vi "ZC_biaoqian.vi"(7 "LabVIEW Web Service Request":refnum<class "Web Request.lvclass"> caption="LabVIEW Web服务请求", 8 "key":string, 9 "number":string, 10 "action":string, 11 "id":string) -> (6 "error":errorcluster)   [LabVIEW 2017]
uses:
  <vilib>/wsapi/Web Request.lvclass
panel:
  out "postdata":string caption="post数据"
  out "error out":errorcluster caption="错误输出"
  # "Web服务请求输入接线端用于调用“Web服务”选板的VI。除非不需要访问该选板，否则不要在连线板上删除这个输入接线端。"
  # "添加至连线板的每一个其他输入控件，在URL中对应于一个输入。如需在接线端模式输出（默认设置）下包含显示控件，则该显示控件必须与连线板相连。"
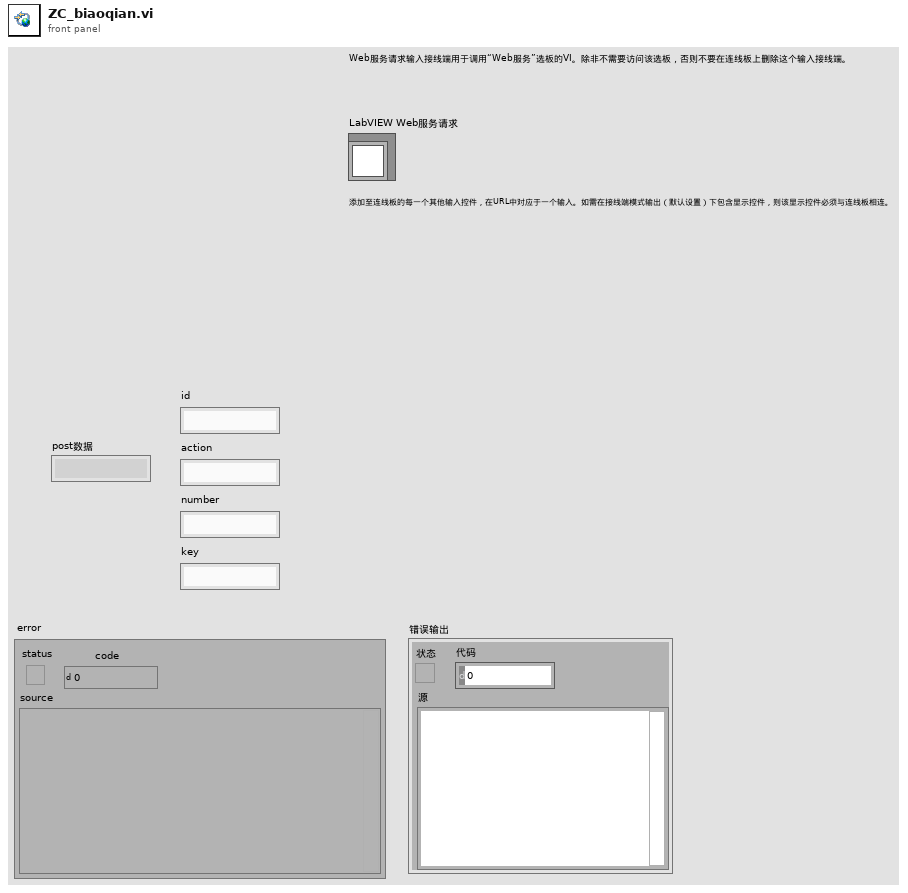
[diagram p1: front panel]
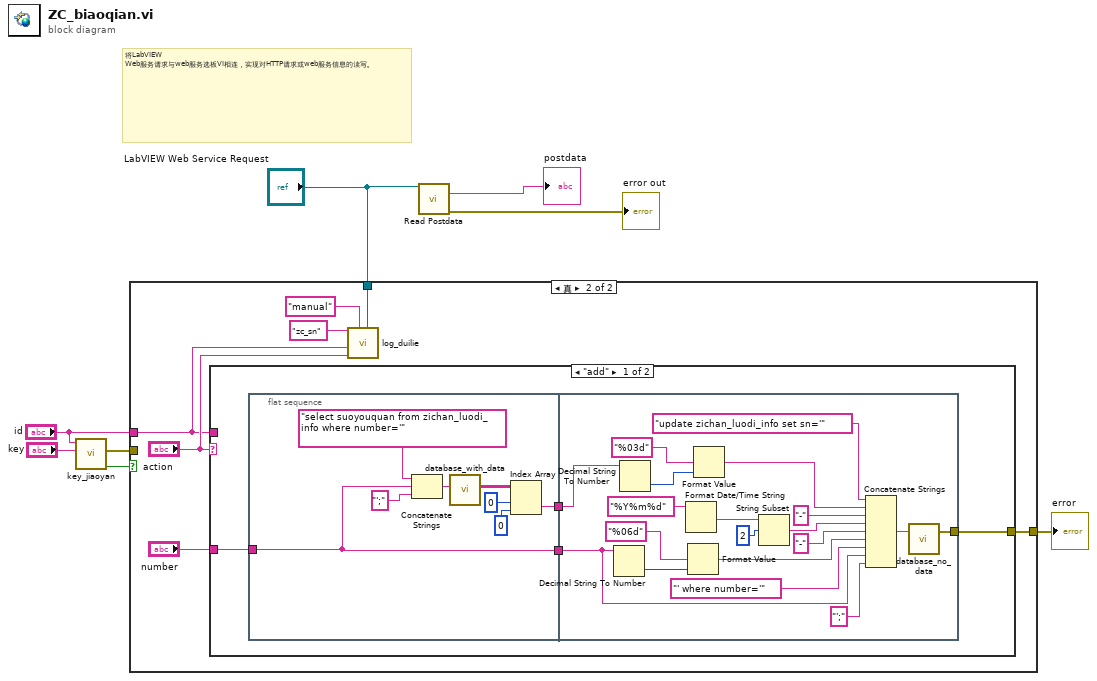
[diagram p0: block diagram]
diagram:
  # "将LabVIEW Web服务请求与web服务选板VI相连，实现对HTTP请求或web服务信息的读写。"
  n1 = call "key_jiaoyan.vi"("key_client"="key", "gonghao"="id") -> ("jy"=w3:bool, "error"=w2:errorcluster)  [unwired: 8 in]
  n2 = case shown="真" w3 {
    tunnel: [w9 w16] -> w7
    tunnel: "LabVIEW Web Service Request" -> [_ w12]
    tunnel: "id" -> [_ w10]
    tunnel: w2 -> [w9 _]
    frame False {
    }
    frame True {
      n3 = case shown="\"add\"" "action" {
        tunnel: [w20 _] -> w16
        tunnel: w10 -> [_ _]
        tunnel: "number" -> [w18 _]
        frame "add" {
          n4 = flat-sequence {
            tunnel: [w22] -> w19
            tunnel: w18 -> [w21]
            tunnel: [w21] -> w17
            tunnel: [w45] -> w20
            tunnel: w19 -> [w42]
            tunnel: w17 -> [w29]
            frame #0 {
              n5 = Concatenate Strings("select suoyouquan from zichan_luodi_info where number='" ("字符串"), w21, "';" ("字符串")) -> (w24:string)
              n6 = call "database_with_data.vi"("input"=w24) -> ("Data"=w23:string[][])  [unwired: 9 in, 1 out]
              n7 = Index Array(array=w23, index (row)=0 ("索引 (行)"), index (col)=0 ("禁用的索引 (列)")) -> (element=w22:string)
            }
            frame #1 {
              n8 = Decimal String To Number(string=w29) -> (number=w34:i32)  [unwired: 2 in, 1 out]
              n9 = Decimal String To Number(string=w42) -> (number=w43:i32)  [unwired: 2 in, 1 out]
              n10 = Format Date/Time String(time format string (%c)="%Y%m%d" ("时间格式字符串(%c)")) -> (date/time string=w39:string)  [unwired: 2 in]
              n11 = Format Value(format string="%06d" ("格式字符串"), value (0)=w34) -> (output string=w32:string)  [unwired: 1 in]
              n12 = Format Value(format string="%03d" ("格式字符串"), value (0)=w43) -> (output string=w41:string)  [unwired: 1 in]
              n13 = String Subset(string=w39, offset (0)=2 ("偏移量(0)")) -> (substring=w36:string)  [unwired: 1 in]
              n14 = Concatenate Strings("update zichan_luodi_info set sn='" ("格式字符串"), w41, "-" ("字符串"), w36, "-" ("字符串"), w32, "' where number='" ("字符串"), w29, "';" ("字符串")) -> (w46:string)
              n15 = call "database_no_data.vi"("input"=w46) -> ("error"=w45:errorcluster)  [unwired: 2 in]
            }
          }
        }
        frame Default {
        }
      }
      n16 = call "log_duilie.vi"("LabVIEW Web Service Request"=w12, "type"="manual", "action"="action", "user"=w10, "yw"="zc_sn") -> ()  [unwired: 7 in]
    }
  }
  "error" <- w7
  n17 = call <vilib>:"Read Postdata.vi"("LabVIEW Web Service Request"="LabVIEW Web Service Request") -> ("postdata"=→"postdata":string, "error out"=→"error out":errorcluster)  [unwired: 12 in, 1 out]
